vi "SetPrivileges.vi"(8 "error in (no error)":errorcluster, 10 "LoginResponse":cluster{"UserInfo":T1, "PassWordExists？":bool}, 11 "TestBench in":refnum<class "TestBench.lvclass">) -> (0 "error out":errorcluster, 3 "TestBench out":refnum<class "TestBench.lvclass">)   [LabVIEW 2019, in "TestBench.lvlib" / "TestBench.lvclass"]
uses:
  TestBench.lvclass
  UserManagement/UserManagement/UserInfo.ctl
  UserManagement/UserManagement/Permission.ctl
  TestBench.lvclass/TestBench.ctl
  EventRecorder/EventRecorder Messages/RecordEvent Msg/RecordEvent Msg.lvclass/RecordEvent Msg.ctl
  <vilib>/ActorFramework/Message Enqueuer/Message Enqueuer.lvclass/Message Enqueuer.ctl
  <vilib>/ActorFramework/Message Enqueuer/Enqueue.vi
  EventRecorder/EventRecorder Messages/RecordEvent Msg/RecordEvent Msg.lvclass
  C:/Program Files (x86)/National Instruments/LabVIEW 2019/vi.lib/ActorFramework/Message/Message.lvclass
  <vilib>/ActorFramework/Message Priority Queue/Priority Enqueue.vi
  UserManagement/UserManagement/UserManagement.lvclass
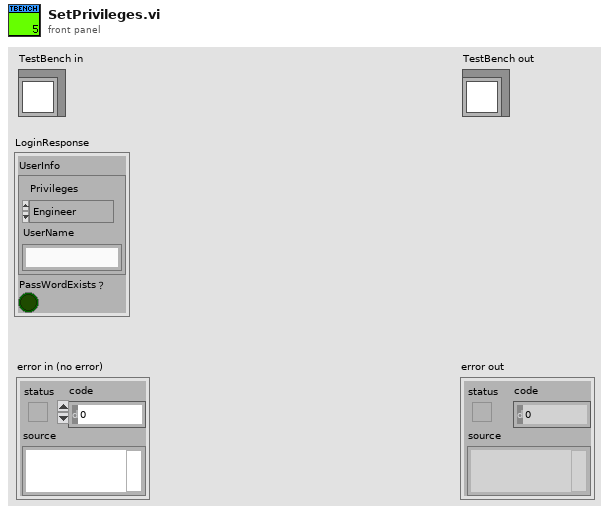
[diagram p1: front panel]
types:
  T1 = typedef "UserManagement.lvlib/UserManagement.lvclass/UserInfo.ctl" = cluster{"Privileges":T2, "UserName":string}
  T2 = typedef "UserManagement.lvlib/UserManagement.lvclass/Permission.ctl" = enum16{"Engineer", "Technical", "Operator"}
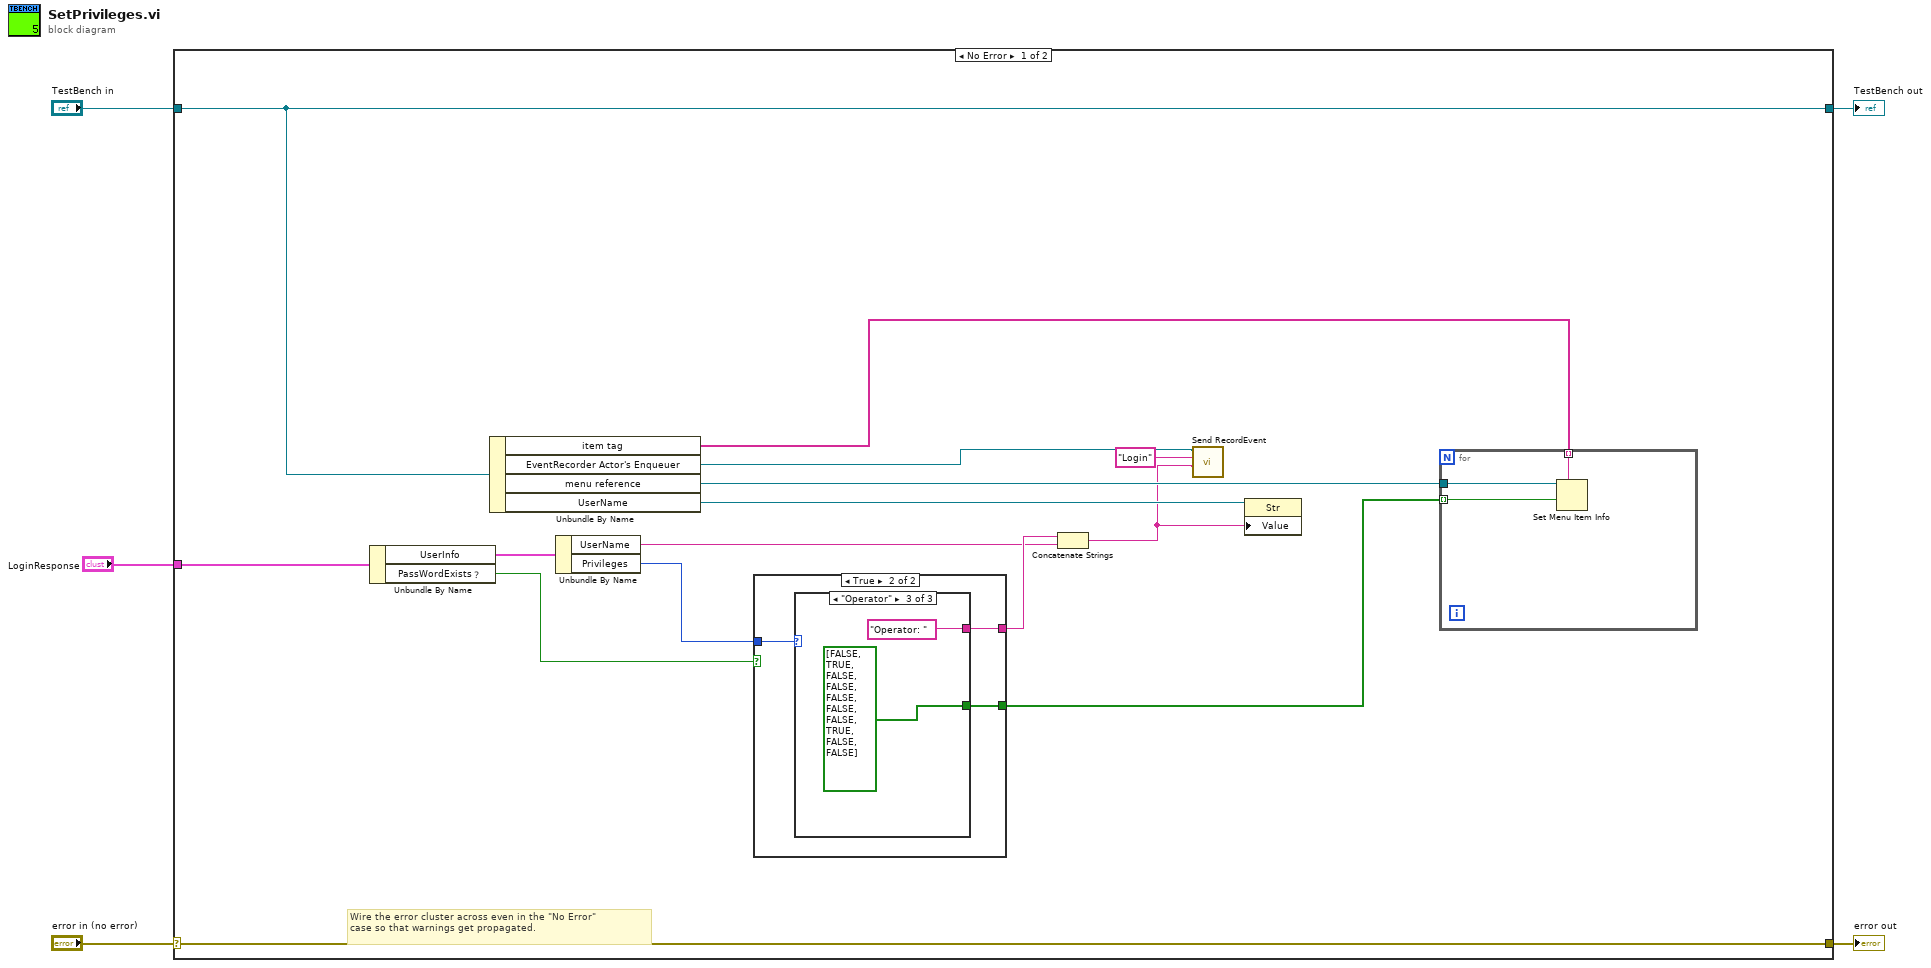
[diagram p0: block diagram]
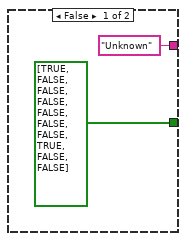
[diagram p2: hidden frame]
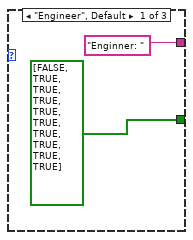
[diagram p3: hidden frame]
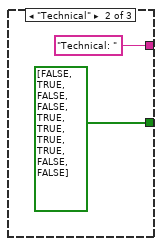
[diagram p4: hidden frame]
diagram:
  n1 = case shown="No Error" "error in (no error)" {
    selector: "error in (no error)" -> [w20 w36]
    tunnel: [w20 w36] -> w4
    tunnel: [w11 w35] -> w2
    tunnel: "TestBench in" -> [w11 w35]
    tunnel: "LoginResponse" -> [w7 _]
    frame No Error {
      # "Wire the error cluster across even in the \"No Error\"\ncase so that warnings get propagated."
      n2 = Unbundle By Name(w7) -> ("UserInfo"=w18:T1, "PassWordExists？"=w15:bool)
      n3 = Unbundle By Name(w11) -> ("item tag"=w6:string[], "EventRecorder Actor's Enqueuer"=w10:refnum<class "Message Enqueuer.lvclass">, "menu reference"=w19:refnum<k9>, "UserName"=w14:refnum<vi>)
      n4 = Unbundle By Name(w18) -> ("UserName"=w12:string, "Privileges"=w17:T2)
      n5 = case shown="True" w15 {
        tunnel: w17 -> [_ w25]
        tunnel: [bool[] [TRUE, FALSE, FALSE, FALSE, FALSE, FALSE, FALSE, TRUE, FALSE, FALSE] w24] -> w16
        tunnel: ["Unknown" w23] -> w13
        frame False {
        }
        frame True {
          n6 = case shown="\"Operator\"" w25 {
            tunnel: [bool[] [FALSE, TRUE, TRUE, TRUE, TRUE, TRUE, TRUE, TRUE, TRUE, TRUE] bool[] [FALSE, TRUE, FALSE, FALSE, TRUE, TRUE, TRUE, TRUE, FALSE, FALSE] bool[] [FALSE, TRUE, FALSE, FALSE, FALSE, FALSE, FALSE, TRUE, FALSE, FALSE]] -> w24
            tunnel: ["Enginner: " "Technical: " "Operator: "] -> w23
            frame "Engineer", Default {
            }
            frame "Technical" {
            }
            frame "Operator" {
            }
          }
        }
      }
      n7 = Concatenate Strings(w13, w12) -> (w8:string)
      n8 = call "Send RecordEvent.vi"("Event Description"=w8, "Event Name"="Login", "Message Enqueuer"=w10) -> ()  [unwired: 7 in, 2 out]
      n9 = property class="Str"(reference=w14, "Value"=w8) -> ()  [unwired: 1 in, 2 out]
      n10 = for {
        tunnel: w19 -> [w34]
        tunnel: w6 -> [w33] mode=indexing
        tunnel: w16 -> [w32] mode=indexing
        n11 = Set Menu Item Info(7:w33, 9:w32, 11:w34) -> ()  [unwired: 4 in, 2 out]
      }
    }
    frame Error {
    }
  }
  "error out" <- w4
  "TestBench out" <- w2
